vi "CloseLog.vi"(8 "error in (no error)":errorcluster, 11 "EventLoggerData out 4":T1) -> (0 "error out":errorcluster, 3 "EventLoggerData out 3":T1)   [LabVIEW 2019, in "EventLogger.lvlib"]
uses:
  EventLogger.lvlib
  Cluster - EventLoggerData.ctl
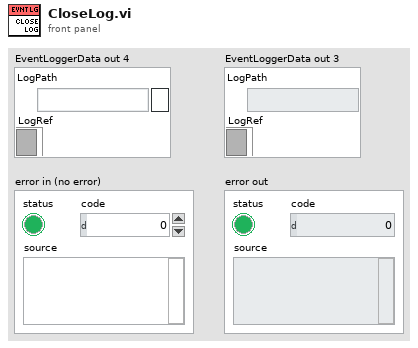
[diagram p1: front panel]
types:
  T1 = typedef "EventLogger.lvlib/Cluster - EventLoggerData.ctl" = cluster{"LogPath":path, "LogRef":refnum<file>}
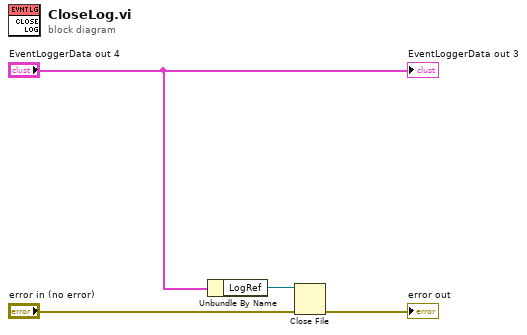
[diagram p0: block diagram]
diagram:
  n1 = Unbundle By Name("EventLoggerData out 4") -> ("LogRef"=w1:refnum<file>)
  n2 = Close File(refnum=w1, error in="error in (no error)") -> (error out=→"error out":errorcluster)  [unwired: 1 out]
  "EventLoggerData out 3" <- "EventLoggerData out 4"
